vi "Dialog Strings.vi"() -> ()   [LabVIEW 2020, in "Output Sequencer.lvlib" / "Settings UI.lvclass"]
uses:
  Settings UI.lvclass
panel:
  in  "Plugin URL":string="https://github.com/ni/niflexlogger-plugins/tree/main/PDK%20plugins/Output%20Sequencer"
  in  "Actions Updated Message":string="The following step(s) have \"Go to\" actions which reference a step that has\nmoved. All of these actions have been updated to point to the new step\nnumbers for their respective steps. Please verify any changed behavior.\n\nAffected step(s):\n"
  in  "Actions Updated Title":string="Actions Updated"
  in  "Actions Removed Message":string="The following step(s) have \"Go to\" actions which reference a step that has\nbeen removed. All of these actions have been updated back to default\n(an empty action, which proceeds to the next step). Please verify any\nchanged behavior.\n\nAffected step(s):\n"
  in  "Actions Removed Title":string="Actions Removed"
  in  "Import Error":string="Import Error"
  in  "Export Error":string="Export Error"
  in  "Expression Error":string="Expression Error"
  in  "Export Exists":string="%s already exists.\n\nWould you like to replace it?"
  in  "Import/Export Label":string="FlexLogger sequence files"
  in  "Revert Message":string="This will revert back to the settings applied to the running plug-in.\nAny pending changes will be lost.\n\nAre you sure you want to revert?"
  in  "Revert Title":string="Confirm revert"
  in  "Apply Message":string="This will apply your pending changes to the running plug-in.\nThis cannot be undone.\n\nAre you sure you want to apply your changes?"
  in  "Apply Title":string="Confirm apply"
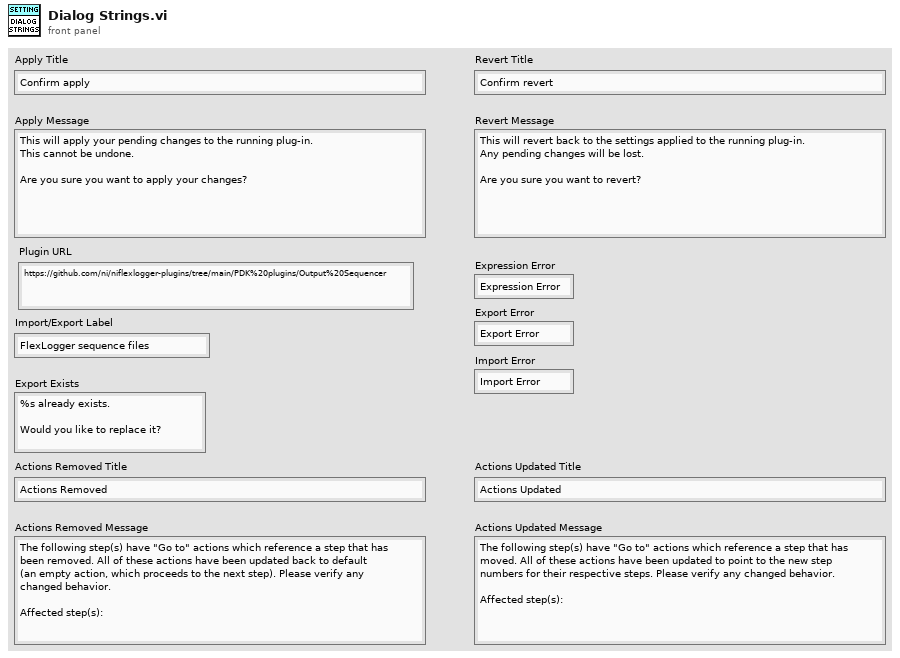
[diagram p1: front panel]
diagram:
